vi "parsePacket.vi"(7 "APRS Packet":string) -> (0 "Token String":string, 1 "Token String":bool, 2 "Altitude":dbl, 3 "Altitude":bool)   [LabVIEW 2012]
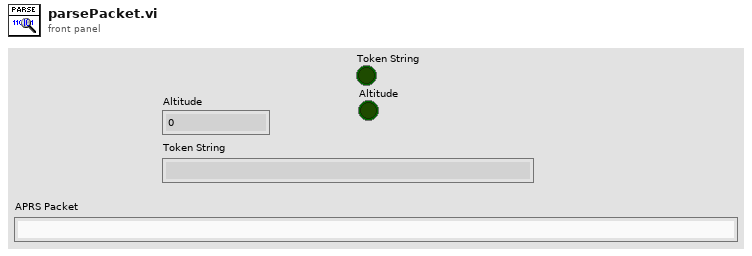
[diagram p1: front panel]
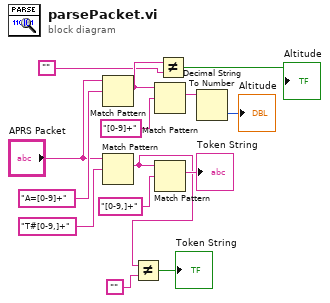
[diagram p0: block diagram]
diagram:
  n1 = Match Pattern(string="APRS Packet", regular expression="A=[0-9]+") -> (match substring=w6:string)  [unwired: 1 in, 3 out]
  n2 = Match Pattern(string="APRS Packet", regular expression="T#[0-9,]+") -> (match substring=w3:string)  [unwired: 1 in, 3 out]
  n3 = Not Equal?(x=w3, y="") -> (x != y?=→"Token String":bool)
  n4 = Match Pattern(string=w6, regular expression="[0-9]+") -> (match substring=w12:string)  [unwired: 1 in, 3 out]
  n5 = Match Pattern(string=w3, regular expression="[0-9,]+") -> (match substring=→"Token String":string)  [unwired: 1 in, 3 out]
  n6 = Not Equal?(x=w6, y="") -> (x != y?=→"Altitude":bool)
  n7 = Decimal String To Number(string=w12) -> (number=→"Altitude":i32)  [unwired: 2 in, 1 out]
